vi "Preset SERIAL NUMBER.vi"(8 "error in (no error)":errorcluster, 10 "SERIAL number":string, 11 "VISA Refnum in":refnum<visa-resource-name>) -> (0 "error out":errorcluster, 3 "VISA Refnum out":refnum<visa-resource-name>)   [LabVIEW 2025, in "Chroma 19052.lvlib"]
uses:
  <instrlib>/Chroma 19052/Chroma 19052.lvlib
panel:
  # "Min 5 char, Max 13 char"
  # "Set SERIAL number"
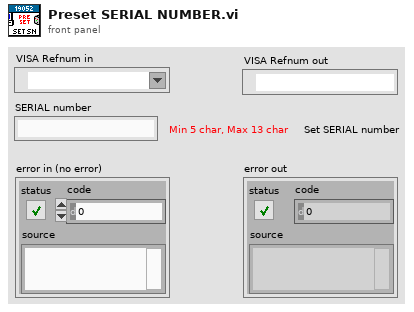
[diagram p1: front panel]
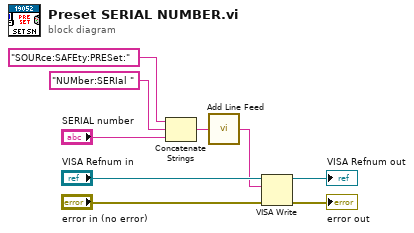
[diagram p0: block diagram]
diagram:
  n1 = Concatenate Strings("SOURce:SAFEty:PRESet:", "NUMber:SERIal ", "SERIAL number") -> (w8:string)
  n2 = call <instrlib>:"Add Line Feed.vi"("Command string"=w8) -> ("Concatenated string"=w1:string)  [unwired: 4 in]
  n3 = VISA Write(VISA resource name="VISA Refnum in", write buffer=w1, error in (no error)="error in (no error)") -> (VISA resource name out=→"VISA Refnum out":refnum<visa-resource-name>, error out=→"error out":errorcluster)  [unwired: 1 out]
